vi "Serialize - JSON.vi"(8 "error in":errorcluster, 11 "Data in":refnum<class "Data.lvclass">) -> (0 "error out":errorcluster, 2 "Serialized JSON":string, 3 "Data out":refnum<class "Data.lvclass">)   [LabVIEW 2014, in "Base Data Class.lvlib" / "Data.lvclass"]
uses:
  Data.lvclass
  Data.lvclass/Data.ctl
  Read Data ID.vi
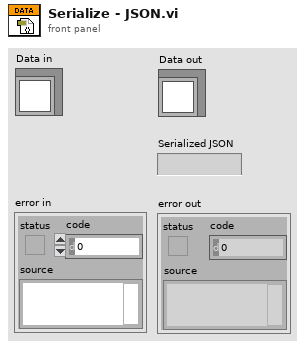
[diagram p1: front panel]
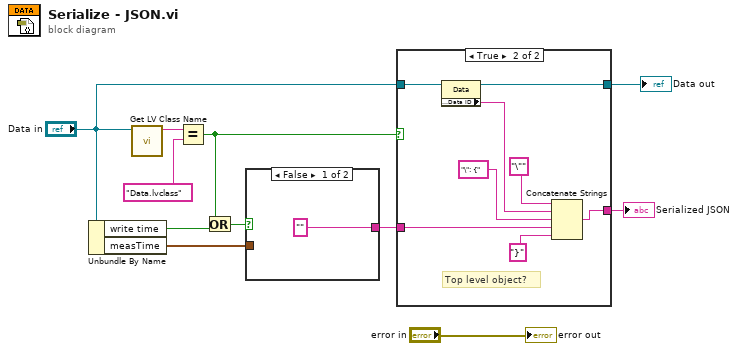
[diagram p0: block diagram]
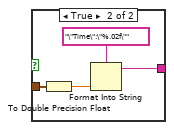
[diagram p3: hidden frame]
diagram:
  n1 = Unbundle By Name("Data in") -> ("write time"=w7:bool, "measTime"=w10:timestamp)
  n2 = call <vilib>:"Get LV Class Name.vi"("object"="Data in") -> ("class name"=w9:string)  [unwired: 9 in, 1 out]
  n3 = Equal?(x=w9, y="Data.lvclass") -> (x = y?=w5:bool)
  n4 = Or(x=w5, y=w7) -> (x .or. y?=w6:bool)
  n5 = case shown="False" w6 {
    tunnel: w10 -> [_ w16]
    tunnel: ["" w14] -> w3
    frame False {
    }
    frame True {
      n6 = To Double Precision Float(number=w16) -> (double precision float=w15:dbl)
      n7 = Format Into String(format string="\"Time\":\"%.02f\"", w15) -> (resulting string=w14:string)  [unwired: 2 in, 1 out]
    }
  }
  n8 = case shown="True" w5 {
    tunnel: "Data in" -> [w17 w26]
    tunnel: w3 -> [w18 w22]
    tunnel: [w18 w20] -> w2
    tunnel: [w17 w19] -> w1
    frame False {
    }
    frame True {
      # "Top level object?"
      n9 = property class="Data"(reference=w26) -> (reference out=w19:refnum<class "Data.lvclass">, "Accessors:Data ID"=w25:string)  [unwired: 1 in, 1 out]
      n10 = Concatenate Strings("\"" ("string"), w25, "\": {" ("string"), w22, "}" ("string")) -> (w20:string)
    }
  }
  "Data out" <- w1
  "Serialized JSON" <- w2
  "error out" <- "error in"
